vi "WebMessaging_Master.vi"() -> (2 "Numeric":i32)   [LabVIEW 2014]
uses:
  <vilib>/httpClient/LabVIEWHTTPClient.lvlib
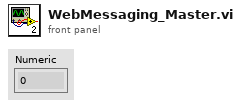
[diagram p1: front panel]
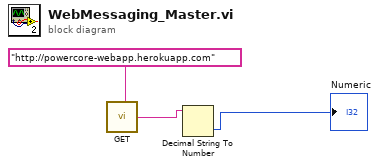
[diagram p0: block diagram]
diagram:
  n1 = call <vilib>:"GET.vi"("url"="http://powercore-webapp.herokuapp.com") -> ("body"=w2:string)  [unwired: 11 in, 3 out]
  n2 = Decimal String To Number(string=w2) -> (number=→"Numeric":i32)  [unwired: 2 in, 1 out]
